vi "Initialize UI Loop.vi"(8 "error in":errorcluster, 11 "UI Data in":T1={"SR Display List"=[], "Filter Cluster"={"Show Resolved"=TRUE, "Show Potentially Resolved"=TRUE, "Show Passoffs"=TRUE, "Show In Collab"=TRUE}, "Exit"=refnum, "Main VI"=refnum, "Sorting"=enum."SR Status", "Message"=refnum, "Legend"=refnum, "Sorting Reference"=refnum, "SR Display List Reference"=refnum, "Filter Cluster Reference"=refnum, "Remove SR"=refnum, "Add SR"=refnum, "Refresh SRs"=refnum} {"SR Display List"."Creation Date" format="%<%x>T"; "SR Display List"."Last Updated" format="%<%x>T"}) -> (0 "error out":errorcluster, 1 "Config File Sort":string, 2 "new user?":bool, 3 "UI Data out":T1={"SR Display List"=[], "Filter Cluster"={"Show Resolved"=TRUE, "Show Potentially Resolved"=TRUE, "Show Passoffs"=TRUE, "Show In Collab"=TRUE}, "Exit"=refnum, "Main VI"=refnum, "Sorting"=enum."SR Status", "Message"=refnum, "Legend"=refnum, "Sorting Reference"=refnum, "SR Display List Reference"=refnum, "Filter Cluster Reference"=refnum, "Remove SR"=refnum, "Add SR"=refnum, "Refresh SRs"=refnum} {"SR Display List"."Creation Date" format="%<%x>T"; "SR Display List"."Last Updated" format="%<%x>T"})   [LabVIEW 2018]
uses:
  Type Defs/UI Loop Data.ctl
  Type Defs/SR Cluster.ctl
  Type Defs/SR Status.ctl
  Type Defs/Filter Cluster.ctl
  Type Defs/Sorting Methods.ctl
  Type Defs/SR Display List Reference.ctl
  Type Defs/FGV States.ctl
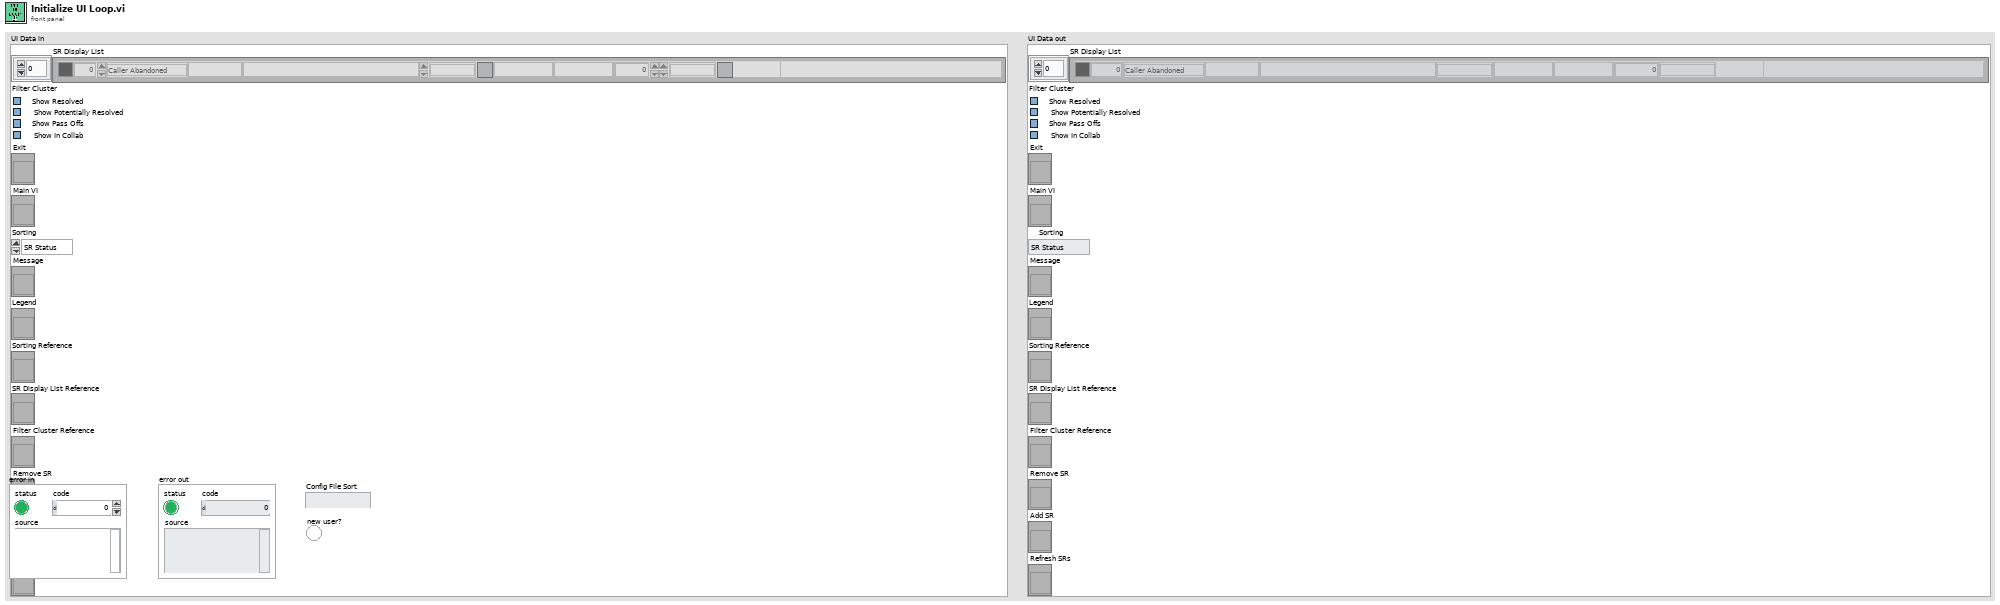
[diagram p1: front panel]
types:
  T1 = typedef "UI Loop Data.ctl" = cluster{"SR Display List":T2[], "Filter Cluster":T4, "Exit":refnum<vi>, "Main VI":refnum<vi>, "Sorting":T5, "Message":refnum<vi>, "Legend":refnum<vi>, "Sorting Reference":refnum<vi>, "SR Display List Reference":T6, "Filter Cluster Reference":refnum<vi>, "Remove SR":refnum<vi>, "Add SR":refnum<vi>, "Refresh SRs":refnum<vi>}
  T2 = typedef "SR Cluster.ctl" = cluster{"Color":u32, "SR Number":i32, "SR Status":T3, "Name":string, "Summary":string, "Last Updated":timestamp, "SR Type":string, "Service Level":string, "Days Open":dbl, "Creation Date":timestamp, "Owner":string, "Note":string}
  T3 = typedef "SR Status.ctl" = enum16{"Caller Abandoned", "Created in Error", "Expired", "Forum Resolved AE", "Forum Resolved Customer", "IN WORK", "IN WORK Collab with AES", "IN WORK Collab with PSE", "IN WORK Collab with SE", "IN WORK Customer Added Note", "IN WORK Escalation", "IN WORK Wait on Customer", "Open", "Potentially Resolved", "Presumed Resolved", "RMA Approved for Return", "RMA Closed", "RMA Closed - DOA", "RMA In Progress", "RMA Open", "RMA Waiting on Customer", "Resolved", "Passed Off"}
  T4 = typedef "Filter Cluster.ctl" = cluster{"Show Resolved":bool, "Show Potentially Resolved":bool, "Show Passoffs":bool, "Show In Collab":bool}
  T5 = typedef "Sorting Methods.ctl" = enum16{"SR Status", "Most Recent", "SR Type", "SR Number", "Days Open", "Urgency"}
  T6 = typedef "SR Display List Reference.ctl" = refnum<vi>
  T7 = typedef "FGV States.ctl" = enum16{"Initialize", "Merge", "Write", "Remove", "Read", "Clear"}
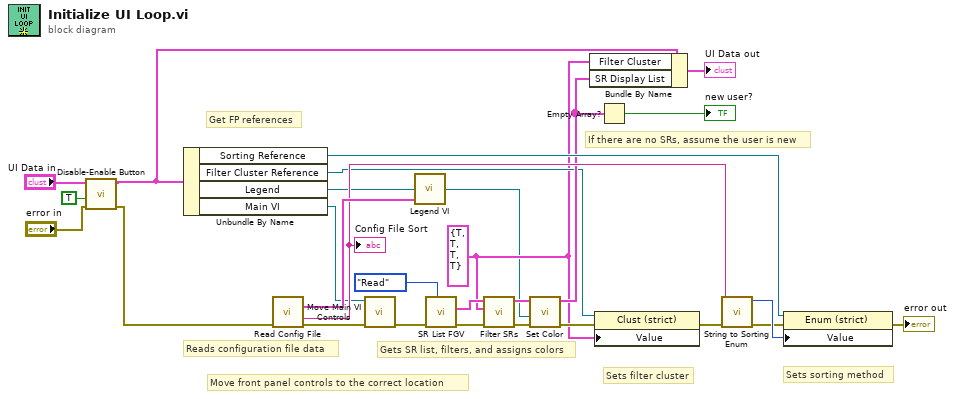
[diagram p0: block diagram]
diagram:
  w7 = T4 {"Show Resolved"=TRUE, "Show Potentially Resolved"=TRUE, "Show Passoffs"=TRUE, "Show In Collab"=TRUE} ("Filter Cluster")
  # "If there are no SRs, assume the user is new"
  # "Sets sorting method"
  # "Sets filter cluster"
  # "Gets SR list, filters, and assigns colors"
  # "Move front panel controls to the correct location"
  # "Reads configuration file data"
  # "Get FP references"
  n1 = call "Disable-Enable Button.vi"("error in"="error in", "Enabled?"=TRUE, "UI Data in"="UI Data in") -> ("error out"=w3:errorcluster, "UI Data out"=w5:T1)  [unwired: 7 in]
  n2 = Unbundle By Name(w5) -> ("Sorting Reference"=w23:refnum<vi>, "Filter Cluster Reference"=w9:refnum<vi>, "Legend"=w8:refnum<vi>, "Main VI"=w10:refnum<vi>)
  n3 = call "Read Config File.vi"("error in (no error)"=w3) -> ("Legend out"=w25:cluster{"Color Box":u32, "String":string}[], "Config File Sort"=w21:string, "error out"=w24:errorcluster)  [unwired: 10 in, 2 out]
  "Config File Sort" <- w21
  n4 = call "Move Main VI Controls.vi"("error in"=w24, "VIRef in"=w10) -> ("error out"=w19:errorcluster)  [unwired: 9 in]
  n5 = call "Legend VI.vi"("Legend in"=w25, "Legend Ref in"=w8) -> ("Legend Ref out"=w1:refnum<vi>)  [unwired: 3 in]
  n6 = call "SR List FGV.vi"("Operation"=FGV_States."Read", "Error In"=w19) -> ("Error Out"=w18:errorcluster, "list out"=w28:T2[])  [unwired: 8 in]
  n7 = call "Filter SRs.vi"("error in"=w18, "Filter Cluster"=w7, "list in"=w28) -> ("error out"=w14:errorcluster, "list out"=w11:T2[])  [unwired: 7 in]
  n8 = call "Set Color.vi"("error in"=w14, "Legend ref"=w1, "list in"=w11) -> ("error out"=w13:errorcluster, "list out"=w12:T2[])  [unwired: 7 in]
  n9 = Bundle By Name(cluster=w5, "Filter Cluster"=w7, "SR Display List"=w12) -> (→"UI Data out":T1)
  n10 = property class="Clust (strict)"(reference=w9, error in=w13, "Value"=w7) -> (error out=w15:errorcluster)  [unwired: 1 out]
  n11 = Empty Array?(array=w12) -> (empty?=→"new user?":bool)
  n12 = call "String to Sorting Enum.vi"("error in"=w15, "string in"=w21) -> ("error out"=w20:errorcluster, "Sorting"=w22:T5)  [unwired: 8 in]
  n13 = property class="Enum (strict)"(reference=w23, error in=w20, "Value"=w22) -> (error out=→"error out":errorcluster)  [unwired: 1 out]
